vi "SetParam.vi"(8 "error in (no error)":errorcluster caption="entrée d'erreur (pas d'erreur)", 10 "polynomial_kernel":T1={"degree"=3, "gamma"="None", "coef0"=1.0}, 11 "Polynomial_kernel.lvclass":refnum<class "Polynomial_kernel.lvclass">) -> (0 "error out":errorcluster caption="sortie d'erreur", 3 "Polynomial_kernel.lvclass":refnum<class "Polynomial_kernel.lvclass">)   [LabVIEW 2020, in "Polynomial_kernel.lvclass"]
doc: "Set Parameters"
uses:
  Polynomial_kernel.lvclass
  Polynomial_kernel.lvclass/Polynomial_kernel.ctl
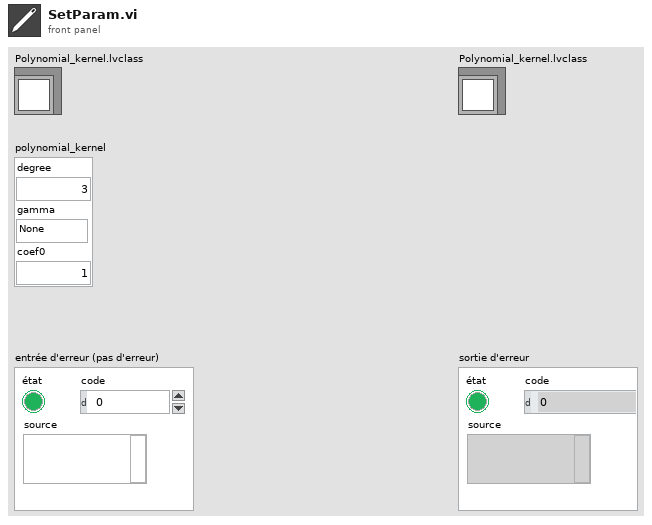
[diagram p1: front panel]
types:
  T1 = cluster{"degree":i32, "gamma":string, "coef0":dbl}
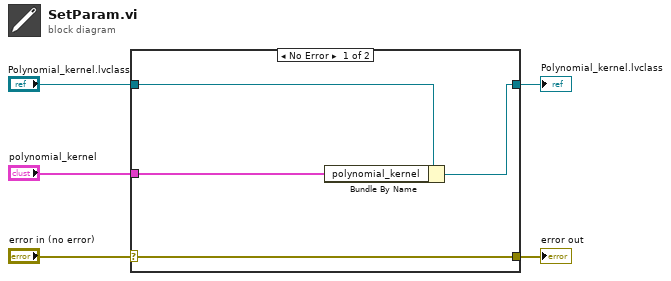
[diagram p0: block diagram]
diagram:
  n1 = case shown="No Error" "error in (no error)" {
    selector: "error in (no error)" -> [w9 w10]
    tunnel: [w9 w10] -> w4
    tunnel: [w7 w11] -> w2
    tunnel: "Polynomial_kernel.lvclass" -> [w8 w11]
    tunnel: "polynomial_kernel" -> [w6 _]
    frame No Error {
      n2 = Bundle By Name(cluster=w8, "polynomial_kernel"=w6) -> (w7:refnum<class "Polynomial_kernel.lvclass">)
    }
    frame Error {
    }
  }
  "error out" <- w4
  "Polynomial_kernel.lvclass" <- w2
